vi "strain_test_v2.vi"() -> ()   [LabVIEW 2014]
uses:
  <vilib>/LabVIEW Targets/FPGA/cRIO/shared/nicrio_ModuleControls/nicrio_cRIO-9237_DataRatesRing.ctl
  <vilib>/LabVIEW Targets/FPGA/cRIO/shared/nicrio_ModuleControls/nicrio_cRIO-9237_ExcitationVoltageRing.ctl
  <vilib>/Platform/TimedLoop/XDataNode/timing_clust.ctl
  <vilib>/Platform/TimedLoop/XDataNode/nitl_modes.ctl
  <vilib>/Platform/TimedLoop/XDataNode/wakeup.ctl
  <vilib>/rvi/FXPMathLib/basic elements/FxpIntAccumulator/subVIs/nifxpmath_IntAccumulator_SimConfig.ctl
  <vilib>/rvi/FXPMathLib/FxpSqrt/subVIs/nifxpmath_Sqrt_SimConfig.ctl
  <vilib>/fxp/LVFixedPointOverflowPolicyTypeDef.ctl
  <vilib>/rvi/Emulation/niFpgaGetClockAttributes.vi
  <vilib>/rvi/Emulation/niFpgaSctlEmulationGetInTimedLoop.vi
  <vilib>/rvi/Emulation/niFpgaEmulationReportErrorSimple.vi
  <vilib>/rvi/Emulation/niFpgaProcessEmulError.vi
  <vilib>/rvi/interface/RandomDataEmulation/nirviRandomDataMultiElementFPGAFIFO.vi
  <instcachedir>/0/nirviRandomDataMultiElementFPGAFIFO_AD0CFC12EF974623A9C2E4184BC062B2.lvgen/nirviRandomDataMultiElementFPGAFIFO_AD0CFC12EF974623A9C2E4184BC062B2_023.vi
  <vilib>/rvi/interface/RandomDataEmulation/niFpgaRandomDataHandleErrors.vi
  <vilib>/rvi/Emulation/niFpgaCriticalErrorInLSC.vi
  <vilib>/rvi/eio/common/nirviEmuTemplatePropertySet_errors.vi
  <vilib>/rvi/eio/common/nirviEmuTemplateMethod_errors.vi
  <vilib>/rvi/Analysis/common/codeGenErrors/XNode/niFpgaXNodeCodeGenErrorHandle.vi
  <vilib>/rvi/FXPMathLib/basic elements/FxpIntAccumulator/simVIs/DllFxpIntAccumulator_sub.vi
  <vilib>/rvi/FXPMathLib/FxpSqrt/simVIs/DllSqrtTemp_sub.vi
  <vilib>/rvi/DataTransferAndStorage/Container/XNode/niFpgaContainer.xnode
  <vilib>/rvi/interface/RandomDataEmulation/nirviRandomDataFpgaMultiElementTemplate.vi
  <vilib>/eio/EIOPropertyNode/EIOPropertyNode.xnode
  <vilib>/eio/EIONode/EIONode.xnode
  <vilib>/rvi/Analysis/measure/butterworth/XNode/niFpgaButterworthFilter.xnode
  <vilib>/rvi/Analysis/measure/dc-rms/XNode/niFpgaDC-RMS.xnode
  <vilib>/Platform/TimedLoop/XDataNode/XDataNode.xnode
  <vilib>/rvi/FXPMathLib/basic elements/FxpIntAccumulator/XNode/nifxpmath_IntAccumulator.xnode
  <vilib>/rvi/FXPMathLib/FxpMul/XNode/nifxpmath_Multiplier.xnode
  <vilib>/rvi/FXPMathLib/FxpSqrt/XNode/nifxpmath_Sqrt.xnode
  <vilib>/rvi/eio/common/nirviEmuTemplatePropertyGet_errors.vi
  <vilib>/rvi/eio/common/nirviEmuTemplatePropertyGet_noerrors.vi
  <vilib>/rvi/eio/common/nirviEmuTemplatePropertySet_noerrors.vi
  <vilib>/Platform/TimedLoop/XDataNode/XDNodeRunTimeDep.lvlib
  <vilib>/rvi/FXPMathLib/sim/FxpSim.dll
panel:
  out "Loop rate (kHz)":fxp<+/-,36,7>
  out "Strain (RMS)":fxp<+,32,44>
  in  "Strain filter coeff.":i32[](array[numeric])=[-850883994, 1909449570, 3794062, -975456236, 2033039520, 4039635]
  out "Force":fxp<+/-,32,10>
  out "Strain":fxp<+/-,42,8>
  out "Fileterd data":fxp<+/-,32,4>
  out "Raw Force":fxp<+/-,32,10>
  in  "S/F coeff":fxp<+/-,41,4>
  out "Raw Strain":fxp<+/-,42,8>
  in  "Reset":bool
  in  "Stop":bool
  out "Mod6/AI2":fxp<+/-,32,4>
  in  "Shunt Cal Enable":bool
  in  "Half-Bridge Enable":bool
  in  "Excitation Voltage":T1 items=["2.5 Volts", "3.3 Volts", "5.0 Volts", "10.0 Volts", "External Excitation"]
  in  "Data Rate":T2=1 items=["50.000 kS/s (NI 9237)"=1, "25.000 kS/s (NI 9237)"=2, "16.667 kS/s (NI 9237)"=3, "12.500 kS/s (NI 9237)"=4, "10.000 kS/s (NI 9237)"=5, "8.333 kS/s (NI 9237)"=6, "7.143 kS/s (NI 9237)"=7, "6.250 kS/s (NI 9237)"=8, "5.556 kS/s (NI 9237)"=9, "5.000 kS/s (NI 9237)"=10, "4.545 kS/s (NI 9237)"=11, "4.167 kS/s (NI 9237)"=12, "3.846 kS/s (NI 9237)"=13, "3.571 kS/s (NI 9237)"=14, "3.333 kS/s (NI 9237)"=15, "3.125 kS/s (NI 9237)"=16, "2.941 kS/s (NI 9237)"=17, "2.778 kS/s (NI 9237)"=18, "2.632 kS/s (NI 9237)"=19, "2.500 kS/s (NI 9237)"=20, "2.381 kS/s (NI 9237)"=21, "2.273 kS/s (NI 9237)"=22, "2.174 kS/s (NI 9237)"=23, "2.083 kS/s (NI 9237)"=24, "2.000 kS/s (NI 9237)"=25, "1.923 kS/s (NI 9237)"=26, "1.852 kS/s (NI 9237)"=27, "1.786 kS/s (NI 9237)"=28, "1.724 kS/s (NI 9237)"=29, "1.667 kS/s (NI 9237)"=30, "1.613 kS/s (NI 9237)"=31]
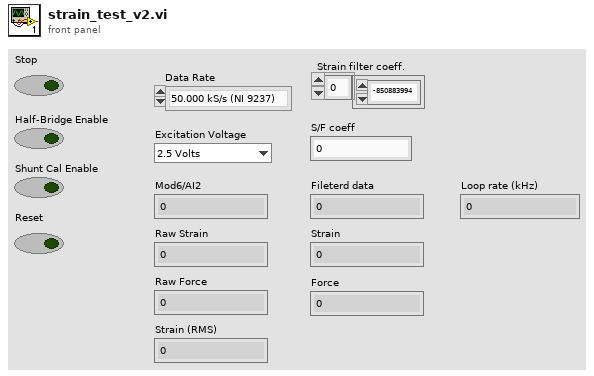
[diagram p1: front panel]
types:
  T1 = typedef "nicrio_cRIO-9237_ExcitationVoltageRing.ctl" = u8
  T2 = typedef "nicrio_cRIO-9237_DataRatesRing.ctl" = u8
  T3 = typedef "XDNodeRunTimeDep.lvlib/timing_clust.ctl" = cluster{"Expected End [f-1]":u64, "Actual End [f-1]":u64, "Finished Late? [f-1]":bool, "Expected End [i-1]":u64, "Actual End [i-1]":u64, "Finished Late? [i-1]":bool, "Expected Start [i]":u64, "Actual Start [i]":u64, "Expected Start [f]":u64, "Actual Start [f]":u64, "Source Name":string, "Structure Name":string, "Period":i64, "Deadline":i64, "Offset":i64, "Start":i64, "Priority":i32, "Timeout":i32, "Mode":T4, "Wakeup Reason":T5, "Error":errorcluster, "Source Type":string, "Secondary Source Type":string, "Global End Time":u64, "Global Start Time":u64, "Frame Duration":u64, "Iteration Duration":u64, "Assigned CPU":i32, "I/O Scan Engine Mode":u32}
  T4 = typedef "XDNodeRunTimeDep.lvlib/nitl_modes.ctl" = enum32{"No Change", "Process missed periods, maintain original phase", "Discard missed periods, maintain original phase", "Process missed periods, ignore original phase", "Discard missed periods, ignore original phase"}
  T5 = typedef "XDNodeRunTimeDep.lvlib/wakeup.ctl" = enum32{"Normal", "Aborted", "Asynchronous wakeup", "Timing source error", "Timed loop error", "Timeout"}
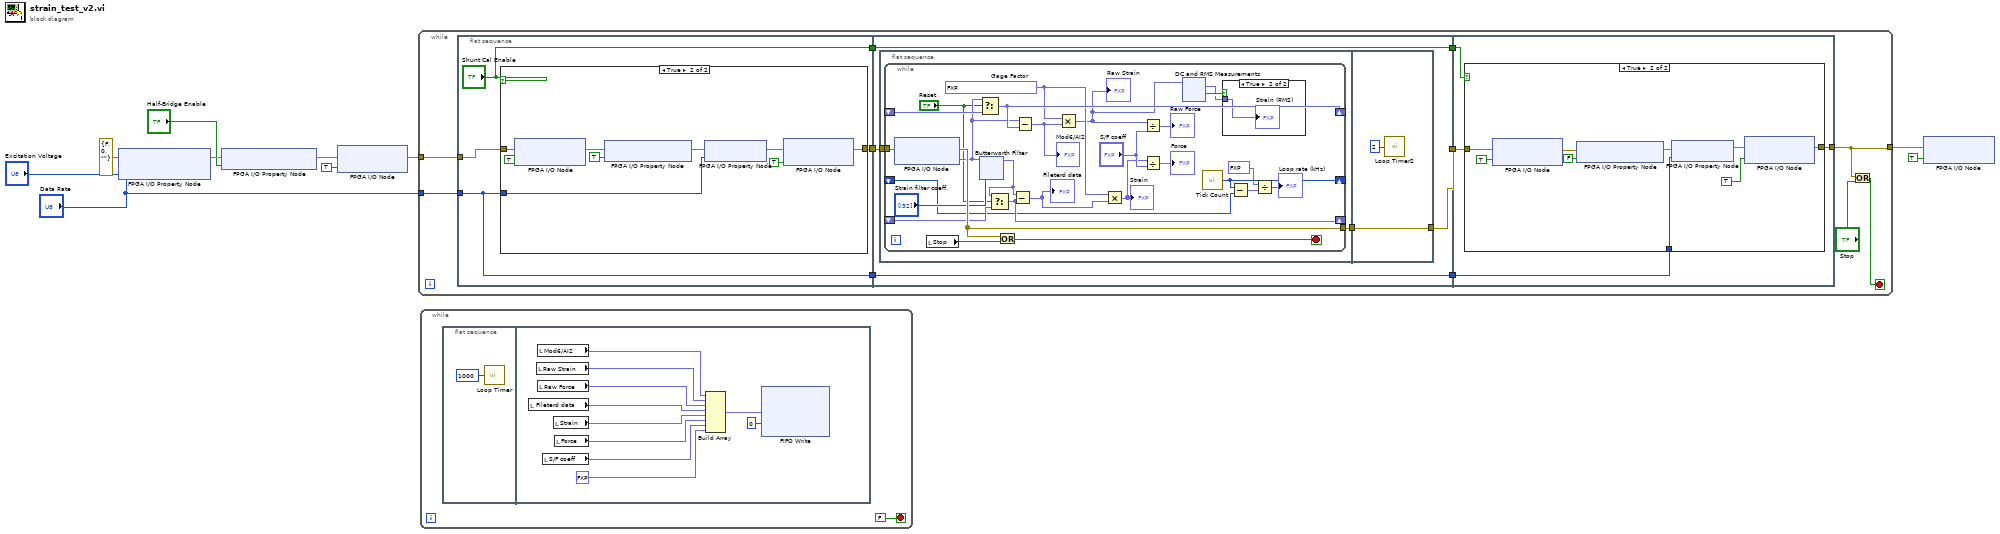
[diagram p0: block diagram]
diagram:
  n1 = xnode "FPGA I/O Property Node"("error in"=errorcluster {"status"=FALSE, "code"=0, "source"=""}, "Data Rate"="Data Rate", "Excitation Voltage"="Excitation Voltage") -> ("error out"=w7:errorcluster)  [unwired: 1 in, 1 out]
  n2 = xnode "FPGA I/O Property Node"("error in"=w7, "Half-Bridge Enable"="Half-Bridge Enable") -> ("error out"=w6:errorcluster)  [unwired: 1 in, 1 out]
  n3 = xnode "FPGA I/O Node"("error in"=w6, "Mod6/Start"=TRUE) -> ("error out"=w4:errorcluster)  [unwired: 1 in, 1 out]
  n4 = while {
    tunnel: w4 -> [w21]
    tunnel: "Data Rate" -> [w20]
    tunnel: [w12] -> w2
    stop <- w13 stop-if-true
    n5 = flat-sequence {
      tunnel: w21 -> [w25]
      tunnel: w20 -> [w24]
      tunnel: [w24] -> w19
      tunnel: ["Shunt Cal Enable"] -> w18
      tunnel: [w22] -> w17
      tunnel: w19 -> [w38]
      tunnel: w18 -> [w39]
      tunnel: w17 -> [w40]
      tunnel: [w39] -> w16
      tunnel: [w37] -> w15
      tunnel: [w38] -> w14
      tunnel: w16 -> [w221]
      tunnel: w15 -> [w220]
      tunnel: w14 -> [w219]
      tunnel: [w218] -> w12
      frame #0 {
        n6 = case shown="True" "Shunt Cal Enable" {
          tunnel: w25 -> [w26 w33]
          tunnel: w24 -> [_ w31]
          tunnel: [w26 w28] -> w22
          frame False {
          }
          frame True {
            n7 = xnode "FPGA I/O Node"("error in"=w33, "Mod6/Stop"=TRUE) -> ("error out"=w34:errorcluster)  [unwired: 1 in, 1 out]
            n8 = xnode "FPGA I/O Property Node"("error in"=w34, "Shunt Cal Enable"=TRUE) -> ("error out"=w32:errorcluster)  [unwired: 1 in, 1 out]
            n9 = xnode "FPGA I/O Property Node"("error in"=w32, "Data Rate"=w31) -> ("error out"=w30:errorcluster)  [unwired: 1 in, 1 out]
            n10 = xnode "FPGA I/O Node"("error in"=w30, "Mod6/Start"=TRUE) -> ("error out"=w28:errorcluster)  [unwired: 1 in, 1 out]
          }
        }
      }
      frame #1 {
        n11 = flat-sequence {
          tunnel: w40 -> [w42]
          tunnel: [w41] -> w36
          tunnel: [w217] -> w37
          tunnel: w36 -> [w217]
          frame #0 {
            n12 = while {
              tunnel: w42 -> [w69]
              tunnel: [w67] -> w41
              shift-right: [w65] -> _
              shift-left: _ -> [w66]
              shift-right: [w61] -> _
              shift-left: _ -> [w62]
              shift-right: [w48] -> _
              shift-left: _ -> [w49]
              stop <- w54 stop-if-true
              w59 = fxp<+,20,2> 2.115001678466797  # Gage Factor
              n13 = xnode "FPGA I/O Node"("error in"=w69) -> ("error out"=w67:errorcluster, "Mod6/AI2"=w63:fxp<+/-,24,-4>)  [unwired: 1 in, 1 out]
              n14 = local read "Stop"() -> (w68:bool)
              n15 = xnode "Butterworth Filter"("input data"=w63, "scaled coefficients"="Strain filter coeff.") -> ("output data"=w60:fxp<+/-,28,0>)  [unwired: 1 in]
              n16 = Select(t=w63, s="Reset", f=w66) -> (s? t:f=w65:fxp<+/-,24,-4>)
              n17 = Select(t=w60, s="Reset", f=w62) -> (s? t:f=w61:fxp<+/-,28,0>)
              n18 = Or(x=w67, y=w68) -> (x .or. y?=w54:bool)
              n19 = Subtract(x=w60, y=w61) -> (x-y=w58:fxp<+/-,32,16>)
              "Fileterd data" <- w58
              n20 = Subtract(x=w63, y=w65) -> (x-y=w64:fxp<+/-,25,-3>)
              "Mod6/AI2" <- w64
              n21 = Multiply(x=w59, y=w64) -> (x*y=w46:fxp<+/-,41,6>)
              "Raw Strain" <- w46
              n22 = Multiply(x=w59, y=w58) -> (x*y=w56:fxp<+/-,41,6>)
              "Strain" <- w56
              n23 = Divide(x=w46, y="S/F coeff") -> (x/y=→"Raw Force":fxp<+/-,64,44>)
              n24 = Divide(x=w56, y="S/F coeff") -> (x/y=→"Force":fxp<+/-,64,44>)
              n25 = xnode ("DC and RMS Measurements")("input data"=w46) -> ("RMS"=w50:fxp<+,32,6>, "output valid"=w51:bool)  [unwired: 1 in, 1 out]
              n26 = call "Tick Count"() -> ("Tick Count(uSec)"=w48:u32)
              n27 = case shown="True" w51 {
                tunnel: w50 -> [_ w70]
                frame False {
                }
                frame True {
                  "Strain (RMS)" <- w70
                }
              }
              n28 = Subtract(x=w48, y=w49) -> (x-y=w45:fxp<+/-,32,16>)
              n29 = Divide(x=fxp<+,7,10> 1000.0, y=w45) -> (x/y=→"Loop rate (kHz)":fxp<+/-,40,27>)
            }
          }
          frame #1 {
            n30 = call "Loop Timer2"("Count(uSec)"=u32 2) -> ()  [unwired: 1 out]
          }
        }
      }
      frame #2 {
        n31 = case shown="True" w221 {
          tunnel: w220 -> [w222 w230]
          tunnel: w219 -> [_ w226]
          tunnel: [w222 w223] -> w218
          frame False {
          }
          frame True {
            n32 = xnode "FPGA I/O Node"("error in"=w230, "Mod6/Stop"=TRUE) -> ("error out"=w228:errorcluster)  [unwired: 1 in, 1 out]
            n33 = xnode "FPGA I/O Property Node"("error in"=w228, "Shunt Cal Enable"=FALSE) -> ("error out"=w227:errorcluster)  [unwired: 1 in, 1 out]
            n34 = xnode "FPGA I/O Property Node"("error in"=w227, "Data Rate"=w226) -> ("error out"=w225:errorcluster)  [unwired: 1 in, 1 out]
            n35 = xnode "FPGA I/O Node"("error in"=w225, "Mod6/Start"=TRUE) -> ("error out"=w223:errorcluster)  [unwired: 1 in, 1 out]
          }
        }
      }
    }
    n36 = Or(x=w12, y="Stop") -> (x .or. y?=w13:bool)
  }
  n37 = while {
    stop <- FALSE stop-if-true
    n38 = flat-sequence {
      frame #0 {
        n39 = call "Loop Timer"("Count(uSec)"=u32 1000) -> ()  [unwired: 1 out]
      }
      frame #1 {
        n40 = local read "Fileterd data"() -> (w240:fxp<+/-,32,4>)
        n41 = local read "Raw Strain"() -> (w242:fxp<+/-,42,8>)
        n42 = local read "Mod6/AI2"() -> (w243:fxp<+/-,32,4>)
        n43 = local read "Raw Force"() -> (w241:fxp<+/-,32,10>)
        n44 = local read "S/F coeff"() -> (w237:fxp<+/-,41,4>)
        n45 = local read "Strain"() -> (w239:fxp<+/-,42,8>)
        n46 = local read "Force"() -> (w238:fxp<+/-,32,10>)
        n47 = Build Array(w243, w242, w241, w240, w239, w238, w237, fxp<+,1,1> 0.0) -> (w235:fxp<+/-,47,10>[])
        n48 = xnode ("FIFO Write")("Element"=w235, "Timeout"=0) -> ()  [unwired: 1 in, 2 out]
      }
    }
  }
  n49 = xnode "FPGA I/O Node"("error in"=w2, "Mod6/Stop"=TRUE) -> ()  [unwired: 1 in, 2 out]
